vi "Close.vi"(8 "error in (no error)":errorcluster, 11 "CCD monitor in":refnum<class "CCD monitor.lvclass">) -> (0 "error out":errorcluster, 3 "CCD monitor out":refnum<class "CCD monitor.lvclass">)   [LabVIEW 2016, in "CCD monitor.lvlib" / "CCD monitor.lvclass"]
uses:
  <userlib>/Common Components/Hardware/Abstract System/Monitor/CCD monitor.lvclass
  <userlib>/Common Components/Hardware/Abstract System/Monitor/CCD monitor.lvclass/CCD monitor.ctl
  <userlib>/Common Components/Hardware/CCD/CCD/CCD.lvclass
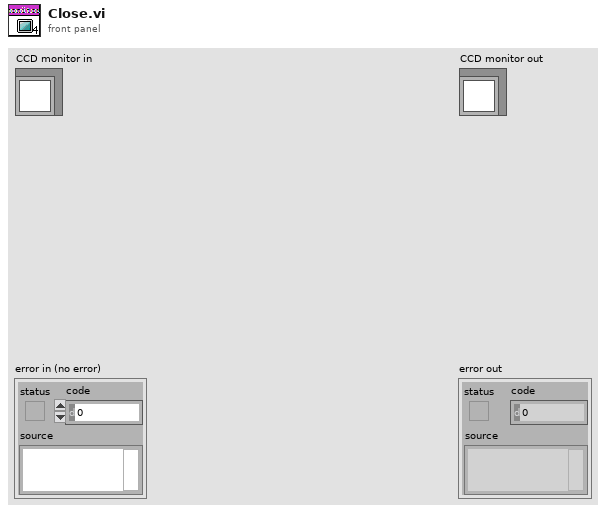
[diagram p1: front panel]
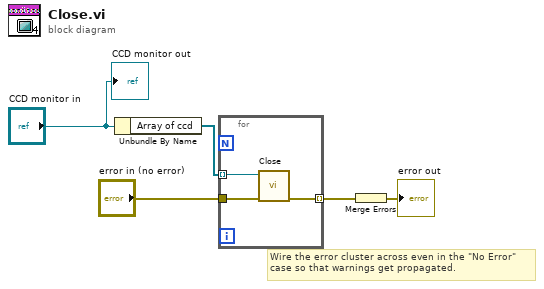
[diagram p0: block diagram]
diagram:
  # "Wire the error cluster across even in the \"No Error\"\ncase so that warnings get propagated."
  n1 = Unbundle By Name("CCD monitor in") -> ("Array of ccd"=w5:refnum<class "CCD.lvclass">[])
  n2 = for {
    tunnel: w5 -> [w8] mode=indexing
    tunnel: "error in (no error)" -> [w7]
    tunnel: [w6] -> w3 mode=indexing
    n3 = call-dynamic "Close.vi"("error in (no error)"=w7, "CCD in"=w8) -> ("error out"=w6:errorcluster)  [unwired: 8 in, 1 out]
  }
  n4 = Merge Errors(w3) -> (→"error out":errorcluster)
  "CCD monitor out" <- "CCD monitor in"
